vi "SQL Execute.vi"(6 "Retries":i32, 8 "error in (no error)":errorcluster, 9 "Return Data (T)":bool=TRUE, 10 "Command Text":string, 11 "ADODB._Connection In":refnum<k7>) -> (0 "error out":errorcluster, 1 "Rows Fetched":i32, 2 "Data":string[][](array[string]), 3 "ADODB._Connection Out":refnum<k7>)   [LabVIEW 2015]
doc: "SQL Execute is a top-level function for performing a SQL query on a database, and if appropriate, getting the rows that are returned by the query. It assumes you have already created an ADO Connection object, which you must wire to this VI's input.\n\nCommand Text is the SQL statement (be sure and terminate it with a semicolon).\nReturn Data is a Boolean, which when TRUE (the default), tells this VI to retrieve data back from the query. Only set this to FALSe if you are sending a SQL command that will not return data (eg, an UPDATE command).\n\nData is a 2-D array of strings which contains the rows returned by the SQL statement.\n\nRows fetched tells you how many rows were returned by the function.\n\nRetries is a integer that lets you specify how many times you wan to retry the SQL command. Normally you shouldn't need this; use it only if you have a very slow DB or the records are being locked out whil you try to execute a SQL command."
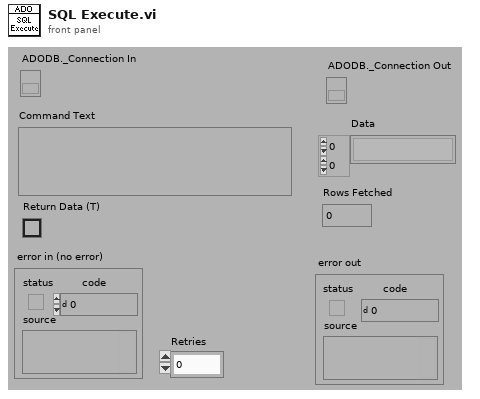
[diagram p1: front panel]
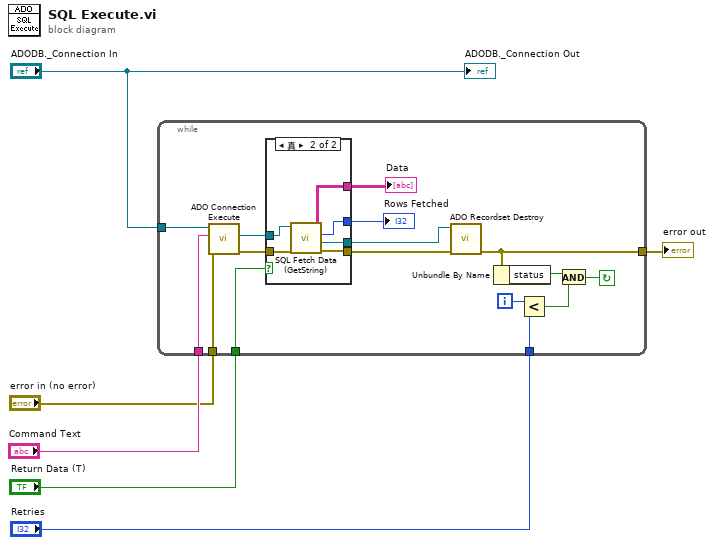
[diagram p0: block diagram]
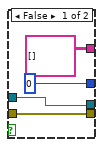
[diagram p2: hidden frame]
diagram:
  n1 = while {
    tunnel: "Retries" -> [w7]
    tunnel: [w12] -> w2
    tunnel: "ADODB._Connection In" -> [w19]
    tunnel: "error in (no error)" -> [w20]
    tunnel: "Command Text" -> [w21]
    tunnel: "Return Data (T)" -> [w22]
    i -> [w10]
    stop <- w8 continue-if-true
    n2 = call <userlib>:"ADO Connection Execute.vi"("error in (no error)"=w20, "CommandText"=w21, "ADODB._Connection In"=w19) -> ("error out"=w18:errorcluster, "RecordSet"=w17:refnum<k7>)  [unwired: 6 in, 1 out]
    n3 = case shown="真" w22 {
      tunnel: w18 -> [w26 w32]
      tunnel: w17 -> [w25 w31]
      tunnel: [0 ("Rows Fetched") w30] -> w16
      tunnel: [string[][] [] ("Data") w29] -> w15
      tunnel: [w26 w28] -> w14
      tunnel: [w25 w27] -> w13
      frame False {
      }
      frame True {
        n4 = call <userlib>:"SQL Fetch Data (GetString).vi"("error in (no error)"=w32, "ADODB._Recordset In"=w31) -> ("error out"=w28:errorcluster, "ADODB._Recordset Out"=w27:refnum<k7>, "Rows Fetched"=w30:i32, "Data"=w29:string[][])  [unwired: 6 in]
      }
    }
    "Data" <- w15
    "Rows Fetched" <- w16
    n5 = call <userlib>:"ADO Recordset Destroy.vi"("error in (no error)"=w14, "ADODB._Recordset In"=w13) -> ("error out"=w12:errorcluster)  [unwired: 9 in]
    n6 = Unbundle By Name(w12) -> ("status"=w11:bool)
    n7 = Less?(x=w10, y=w7) -> (x < y?=w9:bool)
    n8 = And(x=w11, y=w9) -> (x .and. y?=w8:bool)
  }
  "error out" <- w2
  "ADODB._Connection Out" <- "ADODB._Connection In"
